vi "Hatch Immediate.vi"(7 "Description":string, 8 "Command Info In":T2, 11 "Action":T1=enum."Reverse") -> (0 "Command Info Out":T2)   [LabVIEW 2019]
doc: "This template is useful for immediate subsystem actions that do not need deadband filtering\n\nBe sure to right-click and select New from Template and save with a new command name."
uses:
  <vilib>/Rock Robotics/WPI/Framework/Command Status Info.ctl
  <vilib>/Rock Robotics/WPI/Framework/Completion Status.ctl
  <vilib>/Rock Robotics/WPI/Framework/Completion Notifier.ctl
  <vilib>/Rock Robotics/WPI/Solenoid/WPI_SolenoidValue.ctl
  Implementation/Hatch Setpoints.ctl
  Implementation/Hatch Operations.ctl
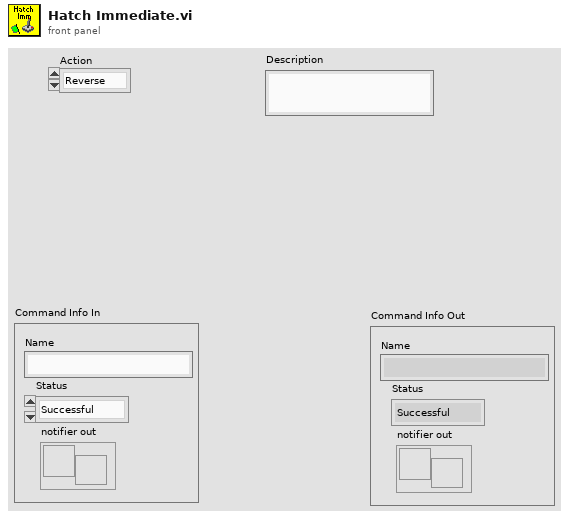
[diagram p1: front panel]
types:
  T1 = typedef "WPI_SolenoidValue.ctl" = enum16{"Off", "On", "Forward", "Reverse"}
  T2 = typedef "Command Status Info.ctl" = cluster{"Name":string, "Status":T3, "notifier out":T4}
  T3 = typedef "Completion Status.ctl" = enum16{"Successful", "Aborted", "Incomplete"}
  T4 = typedef "Completion Notifier.ctl" = refnum<notifier>
  T5 = typedef "Hatch Setpoints.ctl" = cluster{"Operation":T6, "Action":T1}
  T6 = typedef "Hatch Operations.ctl" = enum16{"Reserve", "Read Current", "Immediate", "Hold", "Release"}
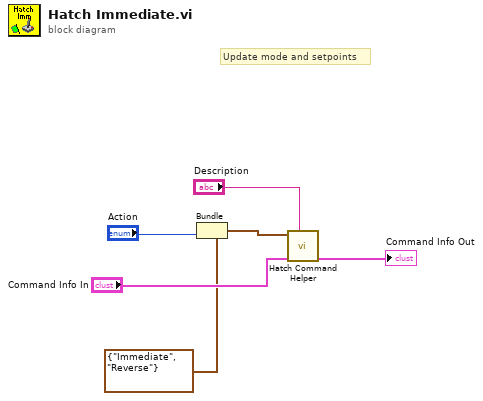
[diagram p0: block diagram]
diagram:
  # "Update mode and setpoints"
  n1 = Bundle(cluster=T5 {"Operation"=enum."Immediate", "Action"=enum."Reverse"} ("SubSystem Data"), "Action"="Action") -> (w2:T5)  [unwired: 1 in]
  n2 = call "Hatch Command Helper.vi"("Description"="Description", "Command Info In"="Command Info In", "SubSystem Data"=w2) -> ("Command Info Out"=→"Command Info Out":T2)  [unwired: 6 in, 2 out]
